vi "DBC-GET-TAG-BY-ID.vi"(8 "error in (no error)":errorcluster, 9 "id":u32 format="%.0x", 11 "dbc in":refnum<class "dbc.lvclass">) -> (0 "error out":errorcluster, 1 "tag":string, 3 "dbc out":refnum<class "dbc.lvclass">)   [LabVIEW 2015, in "dbc.lvclass"]
uses:
  dbc.lvclass
  <vilib>/xnet/xnet.llb/XNET String To IO Name (Frame).vi
  <resource>/objmgr/xnet.rc
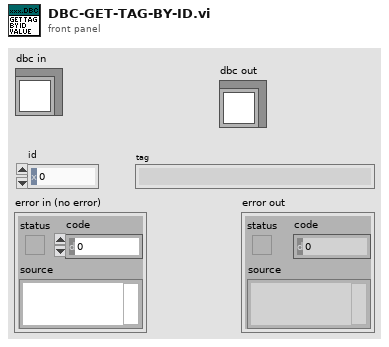
[diagram p1: front panel]
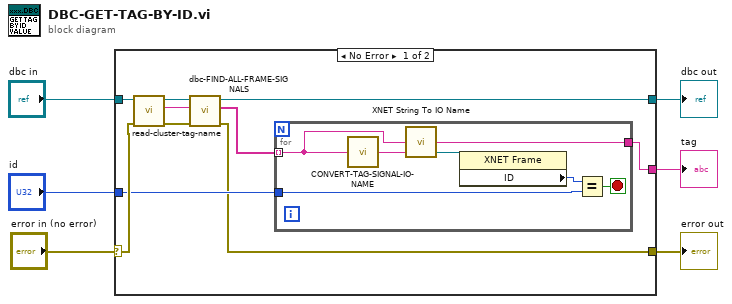
[diagram p0: block diagram]
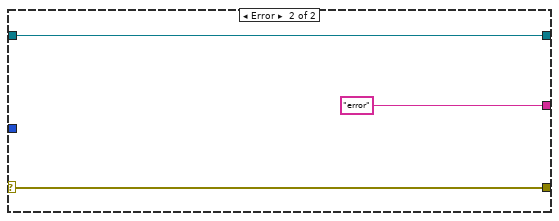
[diagram p2: hidden frame]
diagram:
  n1 = case shown="No Error" "error in (no error)" {
    selector: "error in (no error)" -> [w11 w25]
    tunnel: [w7 w25] -> w5
    tunnel: [w14 w24] -> w3
    tunnel: "dbc in" -> [w16 w24]
    tunnel: "id" -> [w9 _]
    tunnel: [w8 "error"] -> w1
    frame No Error {
      n2 = call "read-cluster-tag-name.vi"("error in (no error)"=w11, "dbc in"=w16) -> ("error out"=w12:errorcluster, "tag.cluster"=w13:string, "dbc out"=w15:refnum<class "dbc.lvclass">)  [unwired: 7 in]
      n3 = call "dbc-FIND-ALL-FRAME-SIGNALS.vi"("error in (no error)"=w12, "tag"=w13, "dbc in"=w15) -> ("error out"=w7:errorcluster, "tag.Array"=w10:string[], "dbc out"=w14:refnum<class "dbc.lvclass">)  [unwired: 6 in]
      n4 = for {
        tunnel: w10 -> [w17] mode=indexing
        tunnel: w9 -> [w20]
        tunnel: [w17] -> w8
        stop <- w19 stop-if-true
        n5 = call "CONVERT-TAG-SIGNAL-IO-NAME.vi"("tag"=w17) -> ("signal"=w18:string)  [unwired: 4 in]
        n6 = call-poly <vilib>:"XNET String To IO Name.vi"("string"=w18) -> ("XNET Frame"=w22:refnum<k21>)  [unwired: 4 out]
        n7 = property class="XNET Frame"(reference=w22) -> ("ID"=w21:u32)  [unwired: 1 in, 2 out]
        n8 = Equal?(x=w21, y=w20) -> (x = y?=w19:bool)
      }
    }
    frame Error {
    }
  }
  "error out" <- w5
  "dbc out" <- w3
  "tag" <- w1
